vi "CAN Frame Output Stream_TEST.vi"() -> ()   [LabVIEW 2020]
doc: "This example demonstrates frame streaming output using an NI-XNET Frame output session. \n\nThis example can run against any input example, assuming you have a properly terminated CAN cable connected to two CAN ports.\n\nIf you have no database aliases on your system, the example automatically loads the nixnet_example database."
uses:
  <vilib>/xnet/xnet.llb/XNET Frame CAN.ctl
  <vilib>/xnet/xnet.llb/XNET Frame Type CAN.ctl
  <vilib>/xnet/xnet.llb/XNET Create Session (Frame Output Stream).vi
  <vilib>/xnet/xnet.llb/XNET Write (Frame CAN).vi
  <resource>/objmgr/xnet.rc
panel:
  in  "data":T1[](array[typedef])=[{"timestamp"=timestamp(0 s since 1904-01-01), "payload"=[120, 2, 78, 32, 188, 102, 119, 136], "identifier"=133, "type"=0, "extended?"=FALSE, "echo?"=FALSE}, {"timestamp"=timestamp(0 s since 1904-01-01), "payload"=[170, 187], "identifier"=67, "type"=0, "extended?"=FALSE, "echo?"=FALSE}, {"timestamp"=timestamp(0 s since 1904-01-01), "payload"=[204, 221, 238, 255, 26, 27, 28, 29], "identifier"=66, "type"=0, "extended?"=FALSE, "echo?"=FALSE}, {"timestamp"=timestamp(0 s since 1904-01-01), "payload"=[65, 66, 67, 68, 69, 70, 71, 71], "identifier"=64, "type"=0, "extended?"=FALSE, "echo?"=FALSE}] {"payload" format="%x"; "timestamp" format="%<%.7X\n%x>T"; "type" items=["CAN Data"=0, "CAN Remote"=1, "CAN Bus Error"=2, "CAN 2.0 Data"=8, "CAN FD Data"=16, "CAN FD+BRS Data"=24, "J1939 Data"=192, "Delay"=224, "Log Trigger"=225, "Start Trigger"=226]; "identifier" format="%08x"}
  in  "CAN Cluster":refnum<k21>="NIXNET_Development.CAN_Cluster"
  in  "Interface Baud Rate":u32=125000
  in  "Select Interface":refnum<k21>="CAN1"
  in  "stop":bool
  # "Overview: Demonstrates the use of the CAN streaming frame output session.\nRequirements: LabVIEW, NI-XNET\nInstructions:\n1. Ensure that you are have connected the selected CAN port to another CAN interface ready to receive data.\n2. Run the VI"
  # "The database's baud rate will be used.  If the :memory: database is used, you must provide a baud rate."
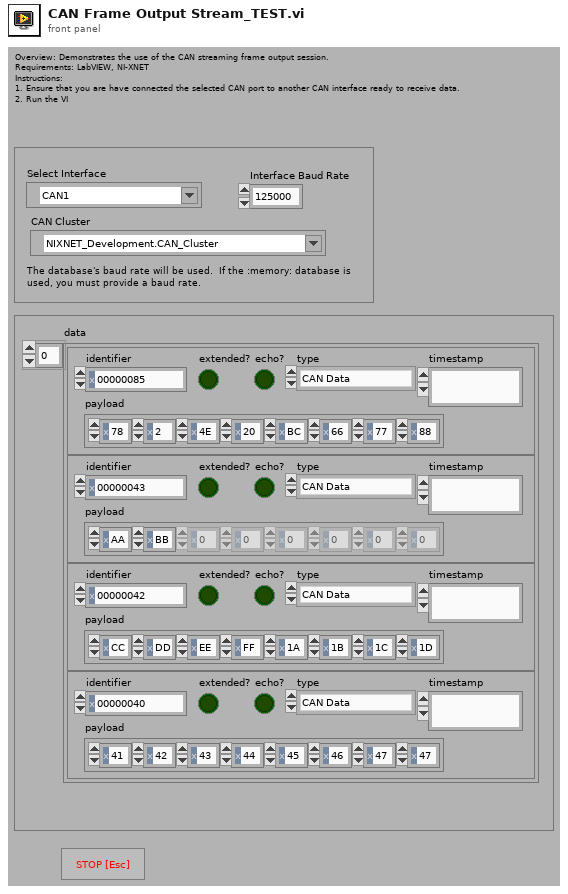
[diagram p1: front panel]
types:
  T1 = typedef "XNET Frame CAN.ctl" = cluster{"timestamp":timestamp, "payload":u8[], "identifier":u32, "type":T2, "extended?":bool, "echo?":bool}
  T2 = typedef "XNET Frame Type CAN.ctl" = u8
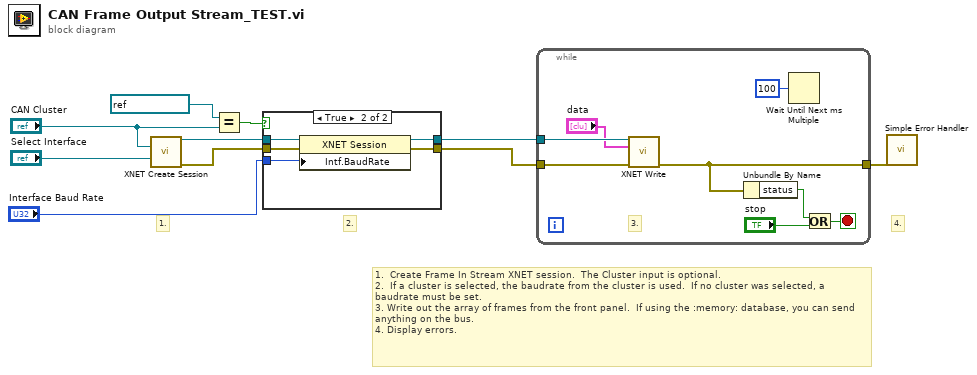
[diagram p0: block diagram]
diagram:
  # "4."
  # "2."
  # "1."
  # "1.  Create Frame In Stream XNET session.  The Cluster input is optional.  \n2.  If a cluster is selected, the baudrate from the cluster is used.  If no cluster was selected, a baudrate must be set.\n3. Write out the array of frames from the front panel.  If using the :memory: database, you can send anything on the bus.\n4. Display errors."
  n1 = call-poly <vilib>:"XNET Create Session.vi"("cluster (:memory:)"="CAN Cluster", "interface"="Select Interface") -> ("session out"=w9:refnum<k21>, "error out"=w5:errorcluster)  [unwired: 1 in, 11 out]
  n2 = Equal?(x=refnum<k21> ":memory:" ("CAN Cluster"), y="CAN Cluster") -> (x = y?=w2:bool)
  n3 = case shown="True" w2 {
    tunnel: w9 -> [w12 w17]
    tunnel: [w12 w16] -> w8
    tunnel: "Interface Baud Rate" -> [_ w15]
    tunnel: [w11 w14] -> w6
    tunnel: w5 -> [w11 w13]
    frame False {
    }
    frame True {
      n4 = property class="XNET Session"(reference=w17, error in=w13, "Intf.BaudRate"=w15) -> (reference out=w16:refnum<k21>, error out=w14:errorcluster)
    }
  }
  n5 = while {
    tunnel: w8 -> [w23]
    tunnel: w6 -> [w22]
    tunnel: [w20] -> w1
    stop <- w25 stop-if-true
    # "3."
    n6 = call-poly <vilib>:"XNET Write.vi"("session in"=w23, "data"="data", "error in (no error)"=w22) -> ("error out"=w20:errorcluster)  [unwired: 12 out]
    n7 = Unbundle By Name(w20) -> ("status"=w24:bool)
    n8 = Wait Until Next ms Multiple(millisecond multiple=u32 100 ("milliseconds to wait")) -> ()  [unwired: 1 out]
    n9 = Or(x=w24, y="stop") -> (x .or. y?=w25:bool)
  }
  n10 = call <vilib>:"Simple Error Handler.vi"("error in (no error)"=w1) -> ()  [unwired: 1 in, 8 out]
